vi "Read Mapped Key.vi"(8 "error in (no error)":errorcluster, 10 "Key":string, 11 "JobReport in":refnum<class "JobReport.lvclass">) -> (0 "error out":errorcluster, 1 "Value":variant, 2 "Key dup":string, 3 "JobReport out":refnum<class "JobReport.lvclass">, 4 "found":bool)   [LabVIEW 2013, in "openCronJob.lvlib" / "JobReport.lvclass"]
uses:
  JobReport.lvclass
  JobReport.lvclass/JobReport.ctl
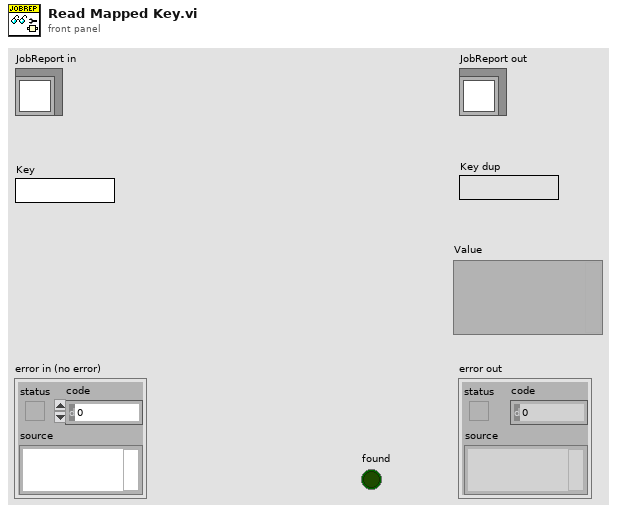
[diagram p1: front panel]
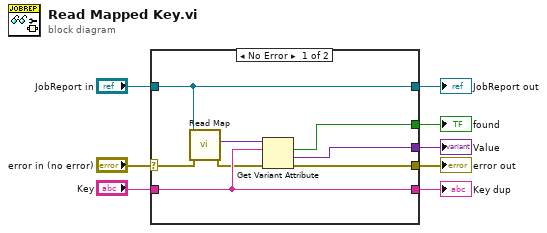
[diagram p0: block diagram]
diagram:
  n1 = case shown="No Error" "error in (no error)" {
    selector: "error in (no error)" -> [w10 w19]
    tunnel: [w12 w19] -> w7
    tunnel: [w11 w18] -> w5
    tunnel: "JobReport in" -> [w11 w18]
    tunnel: [w13 w17] -> w4
    tunnel: "Key" -> [w13 w17]
    tunnel: [w15 _] -> w2
    tunnel: [w14 _] -> w1
    frame No Error {
      n2 = call "Read Map.vi"("error in (no error)"=w10, "JobReport in"=w11) -> ("error out"=w9:errorcluster, "Map"=w16:variant)  [unwired: 7 in, 1 out]
      n3 = Get Variant Attribute(Variant=w16, name=w13, error in=w9) -> (found=w15:bool, value=w14:variant, error out=w12:errorcluster)  [unwired: 1 in, 1 out]
    }
    frame Error {
    }
  }
  "error out" <- w7
  "JobReport out" <- w5
  "Key dup" <- w4
  "found" <- w2
  "Value" <- w1
